vi "Main.vi"() -> ()   [LabVIEW 2012, in "HGF_ApplicationBaseClasses.lvlib" / "HGF_Application.lvclass"]
uses:
  HGF_Application.lvclass
  HGF_BaseClasses/HGF_Factory/HGF_Factory.lvclass
  HGF_BaseClasses/HGF_Event/HGF_Event.lvclass
  HGF_BaseClasses/HGF_Stop/HGF_Stop.lvclass
  HGF_Application.lvclass/HGF_Application.ctl
  HGF_Configuration/HGF_Configuration.lvclass
  HGF_Auxiliary/HGF_Auxiliary.lvlib
  HGF_BaseClasses/HGF_Timing/HGF_Timing.lvclass
  <vilib>/lvdsc/NI_DSC.lvlib
panel:
  in  "HDV":bool
  in  "Alarm and Event Display":refnum<k7>(container)
  in  "read parameters":T1={"Min priority"=0, "Max priority"=1000, "Show Acknowledged alarms?"=FALSE} {"Max priority" max=1000 step=1; "Min priority" max=1000 step=1}
  out "Alarm Summary Data":T2
  out "Time Stamp":timestamp format="%<%H:%M:%S\n%m/%d>T"
  out "Status":string
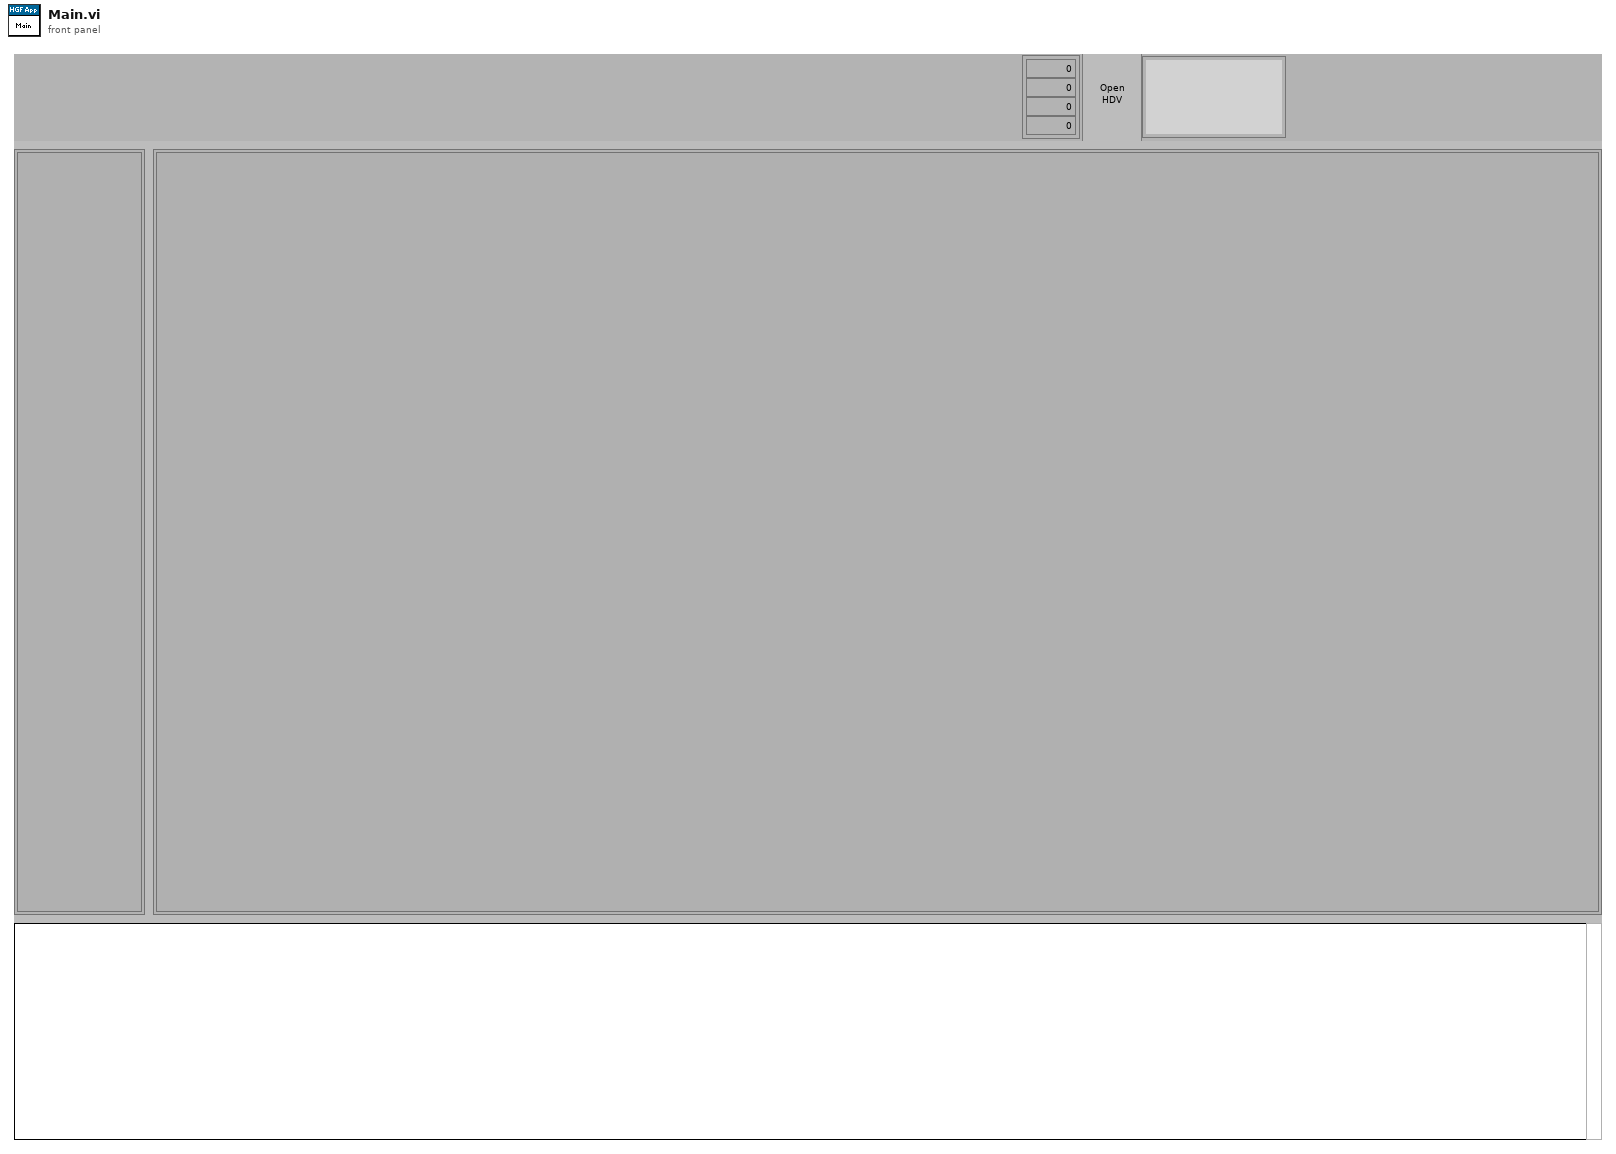
[diagram p1: front panel]
types:
  T1 = cluster{"Min priority":u32, "Max priority":u32, "Show Acknowledged alarms?":bool}
  T2 = cluster{"# active alarms occurrences":i32, "any alarm occurrences?":bool, "# unack alarms occurrences":i32, "any unack alarm occurrences?":bool, "# tags with active alarms":i32, "any tags with alarms?":bool, "# tags with unack alarms":i32, "any tags with unack alarms?":bool}
  T3 = enum32{"invalid app kind", "Development System", "Run Time System", "Student Edition", "Embedded LabVIEW", "Evaluation", "Custom"}
  T4 = cluster{"# active alarms occurrences":i32, "any alarm occurrences?":bool, "# unack alarms occurrences":i32, "any unack alarm occurrences?":bool, "# shared variables with active alarms":i32, "any shared variables with alarms?":bool, "# shared variables with unack alarms":i32, "any shared variables with unack alarms?":bool}
  T5 = cluster{"seconds since 1Jan1904":timestamp, string}
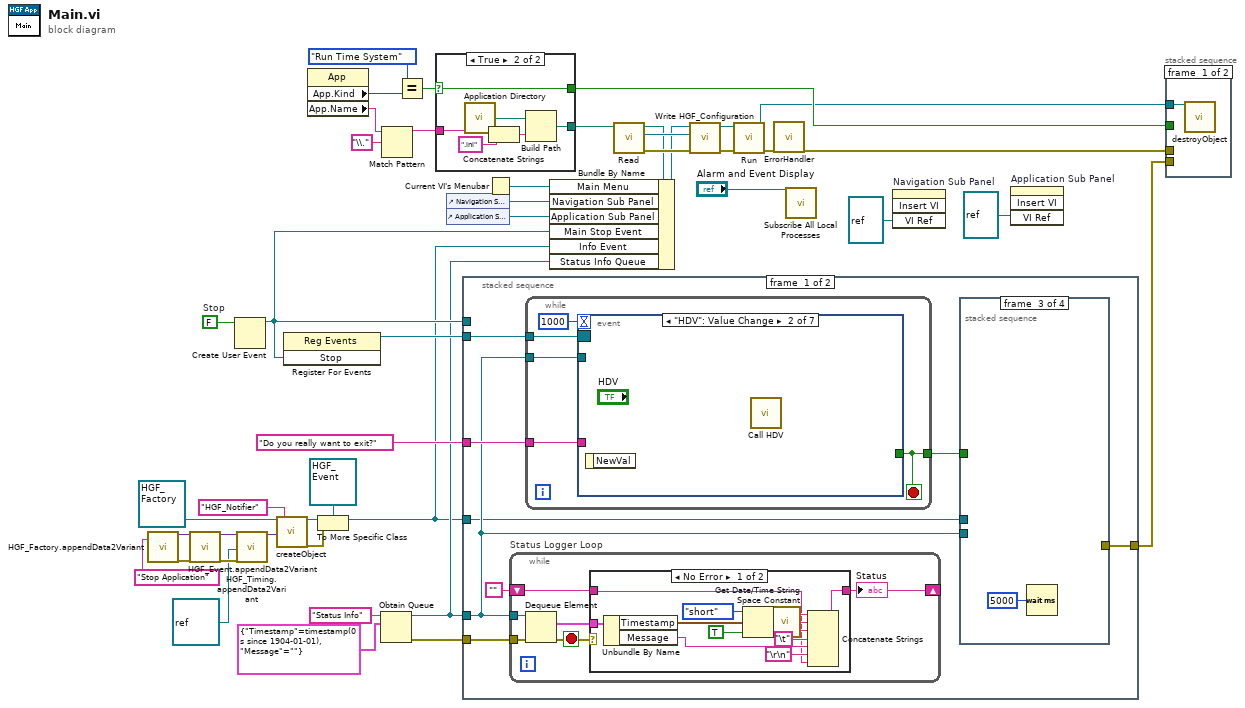
[diagram p0: block diagram]
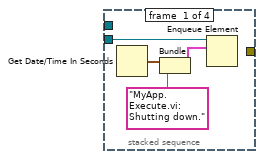
[diagram p2: hidden frame]
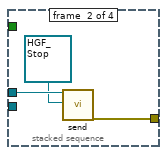
[diagram p3: hidden frame]
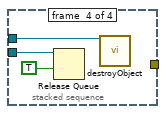
[diagram p4: hidden frame]
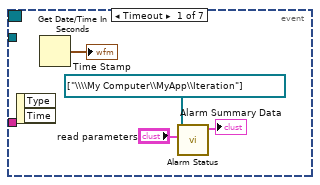
[diagram p6: hidden frame]
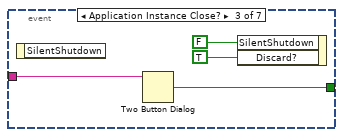
[diagram p7: hidden frame]
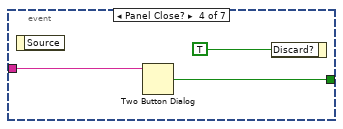
[diagram p8: hidden frame]
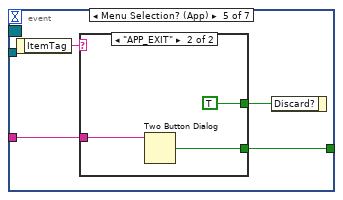
[diagram p9: hidden frame]
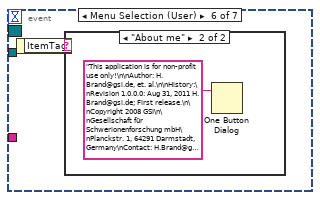
[diagram p11: hidden frame]
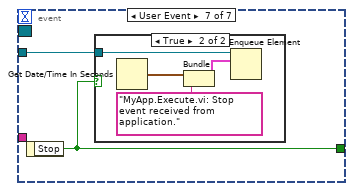
[diagram p13: hidden frame]
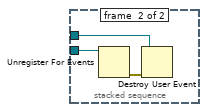
[diagram p15: hidden frame]
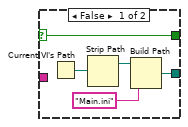
[diagram p16: hidden frame]
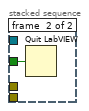
[diagram p17: hidden frame]
diagram:
  w33 = FALSE  # Stop
  n1 = call "HGF_Factory.appendData2Variant.vi"("objectName"="Stop Application") -> ("dup initData"=w20:variant, "error out"=w17:errorcluster)  [unwired: 17 in]
  n2 = call "HGF_Event.appendData2Variant.vi"("initData"=w20, "error in (no error)"=w17) -> ("dup initData"=w19:variant, "error out"=w18:errorcluster)  [unwired: 16 in]
  n3 = Create User Event(user event datatype=w33) -> (user event=w29:refnum<user-event>)  [unwired: 1 in, 1 out]
  n4 = call "HGF_Timing.appendData2Variant.vi"("initData"=w19, "defaultObject"=refnum<class> refnum, "error in (no error)"=w18) -> ("dup initData"=w16:variant)  [unwired: 15 in, 1 out]
  n5 = call "createObject.vi"("HGF_Factory"=refnum<class "HGF_Factory.lvclass"> refnum ("HGF_BaseClasses.lvlib:HGF_Factory.lvclass"), "initializationData"=w16, "className"="HGF_Notifier") -> ("HGF_Object"=w15:refnum<class "HGF_Factory.lvclass">, "error out"=w14:errorcluster)  [unwired: 14 in, 1 out]
  n6 = register-events(w29) -> (reference out=w32:refnum<event-registration>)  [unwired: 2 in, 1 out]
  n7 = property class="App"() -> ("App.Kind"=w37:T3, "App.Name"=w2:string)  [unwired: 2 in, 2 out]
  n8 = To More Specific Class(target class=refnum<class "HGF_Event.lvclass"> refnum ("HGF_BaseClasses.lvlib:HGF_Event.lvclass"), reference=w15, error in=w14) -> (specific class reference=w9:refnum<class "HGF_Event.lvclass">)  [unwired: 1 out]
  n9 = Obtain Queue(name (unnamed)="Status Info", element data type=cluster{"Timestamp":timestamp, "Message":string} {"Timestamp"=timestamp(0 s since 1904-01-01), "Message"=""}) -> (queue out=w10:refnum<queue>, error out=w26:errorcluster)  [unwired: 3 in, 1 out]
  n10 = Match Pattern(string=w2, regular expression="\\.") -> (before substring=w3:string)  [unwired: 1 in, 3 out]
  n11 = Equal?(x=T3."Run Time System" ("Application:Kind"), y=w37) -> (x = y?=w36:bool)
  n12 = case shown="True" w36 {
    selector: w36 -> [w46 w56]
    tunnel: [w47 w54] -> w45
    tunnel: [w46 w56] -> w35
    tunnel: w3 -> [_ w52]
    frame False {
      n13 = Current VI's Path() -> (path=w50:path)
      n14 = Strip Path(path=w50) -> (stripped path=w49:path)  [unwired: 1 out]
      n15 = Build Path(base path=w49, name or relative path="Main.ini") -> (appended path=w47:path)
    }
    frame True {
      n16 = call <vilib>:"Application Directory.vi"() -> ("Application Directory"=w55:path)
      n17 = Concatenate Strings(w52, ".ini" ("name or relative path")) -> (w51:string)
      n18 = Build Path(base path=w55, name or relative path=w51) -> (appended path=w54:path)
    }
  }
  n19 = control-ref of="Navigation Sub Panel"() -> (w8:refnum<vi>)
  n20 = control-ref of="Application Sub Panel"() -> (w7:refnum<vi>)
  n21 = stacked-sequence {
    tunnel: "Do you really want to exit?" ("message") -> [w64 _]
    tunnel: w32 -> [w63 w128]
    tunnel: w29 -> [_ w127]
    tunnel: w10 -> [w60 _]
    tunnel: w26 -> [w62 _]
    tunnel: w9 -> [w58 _]
    tunnel: [w57 _] -> w6
    frame #0 {
      n22 = while "Status Logger Loop" {
        tunnel: w60 -> [w81]
        tunnel: w62 -> [w80]
        shift-right: [w77] -> _
        shift-left: "" -> [w78]
        stop <- w76 stop-if-true
        n23 = Dequeue Element(queue=w81, error in (no error)=w80) -> (element=w79:cluster{"Timestamp":timestamp, "Message":string}, error out=w76:errorcluster)  [unwired: 1 in, 2 out]
        n24 = case shown="No Error" w76 {
          tunnel: w79 -> [w91 _]
          tunnel: w78 -> [w82 w94]
          tunnel: [w83 w94] -> w77
          frame No Error {
            n25 = Unbundle By Name(w91) -> ("Timestamp"=w90:timestamp, "Message"=w86:string)
            n26 = Get Date/Time String(date format (0)=enum16{"short", "long", "abbreviated"}."short", seconds (now)=w90, want seconds? (F)=TRUE) -> (date string=w89:string, time string=w88:string)
            n27 = call <vilib>:"Space Constant.vi"() -> ("String"=w87:string)
            n28 = Concatenate Strings(w89, w87, w88, "\t", w86, "\r\n", w82) -> (w83:string)
          }
          frame Error {
          }
        }
        "Status" <- w77
      }
      n29 = while {
        tunnel: w64 -> [w99]
        tunnel: w63 -> [w98]
        tunnel: [w96] -> w61
        tunnel: w60 -> [w95]
        stop <- w96 stop-if-true
        n30 = event shown="[1] \"HDV\": Value Change" {
          selector: w98 -> [_ _ _ _ _ _ _]
          dyn-events: _ -> [_ _ _ _ _ _ _]
          timeout: 1000 -> [_ _ _ _ _ _ _]
          tunnel: w99 -> [_ _ w105 w109 w113 _ _]
          tunnel: [_ _ w104 w108 w112 _ w120] -> w96
          tunnel: w95 -> [_ _ _ _ _ _ w121]
          event Timeout {
            n31 = event-data() -> ()  [unwired: 1 in, 2 out]
            n32 = Get Date/Time In Seconds() -> (seconds since 1Jan1904=→"Time Stamp":timestamp)
            n33 = call <vilib>:"Alarm Status.vi"("read parameters"="read parameters", "shared variables"=refnum<k21>[] ["\\\\My Computer\\MyApp\\Iteration"]) -> ("alarm summary data"=→"Alarm Summary Data":T4)  [unwired: 8 in, 1 out]
          }
          event "HDV": Value Change {
            n34 = event-data() -> ()  [unwired: 1 in, 1 out]
            n35 = call <vilib>:"Call HDV.vi"() -> ()  [unwired: 14 in, 2 out]
          }
          event Application Instance Close? {
            n36 = event-data() -> ()  [unwired: 1 in, 1 out]
            n37 = Two Button Dialog(message=w105) -> (T button?=w104:bool)  [unwired: 2 in]
            n38 = event-data("SilentShutdown"=FALSE, "Discard?"=TRUE) -> ()  [unwired: 1 in, 1 out]
          }
          event Panel Close? {
            n39 = event-data() -> ()  [unwired: 1 in, 1 out]
            n40 = Two Button Dialog(message=w109) -> (T button?=w108:bool)  [unwired: 2 in]
            n41 = event-data("Discard?"=TRUE) -> ()  [unwired: 1 in, 1 out]
          }
          event Menu Selection? (App) {
            n42 = event-data() -> ("ItemTag"=w114:string)  [unwired: 1 in]
            n43 = case shown="\"APP_EXIT\"" w114 {
              tunnel: w113 -> [_ w117]
              tunnel: [_ w116] -> w112
              tunnel: [_ TRUE] -> w111
              frame "False", Default {
              }
              frame "APP_EXIT" {
                n44 = Two Button Dialog(message=w117) -> (T button?=w116:bool)  [unwired: 2 in]
              }
            }
            n45 = event-data("Discard?"=w111) -> ()  [unwired: 1 in, 1 out]
          }
          event Menu Selection (User) {
            n46 = event-data() -> ("ItemTag"=w118:string)  [unwired: 1 in]
            n47 = case shown="\"About me\"" w118 {
              frame "False", Default {
              }
              frame "About me" {
                n48 = One Button Dialog(message="This application is for non-profit use only!\n\nAuthor: H.Brand@gsi.de, et. al.\n\nHistory:\nRevision 1.0.0.0: Aug 31, 2011 H.Brand@gsi.de; First release.\n\nCopyright 2008 GSI\n\nGesellschaft für Schwerionenforschung mbH\nPlanckstr. 1, 64291 Darmstadt, Germany\nContact: H.Brand@gsi.de or D.Beck@gsi.de\n\nThis file is part of the HGF LVOOP base class library.\n\n    HGF LVOOP base class library is free software: you can redistribute it and/or modify\n    it under the terms of the GNU General Public License as published by\n    the Free Software Foundation, either version 3 of the License, or\n    (at your option) any later version.\n\n    HGF LVOOP base class library is distributed in the hope that it will be useful,\n    but WITHOUT ANY WARRANTY; without even the implied warranty of\n    MERCHANTABILITY or FITNESS FOR A PARTICULAR PURPOSE.  See the\n    GNU General Public License for more details.\n\n    You should have received a copy of the GNU General Public License\n    along with HGF LVOOP base class library.  If not, see http://www.gnu.org/licenses/.") -> ()  [unwired: 1 in, 1 out]
              }
            }
          }
          event User Event {
            n49 = event-data() -> ("Stop"=w120:bool)  [unwired: 1 in]
            n50 = case shown="True" w120 {
              tunnel: w121 -> [_ w125]
              frame False {
              }
              frame True {
                n51 = Get Date/Time In Seconds() -> (seconds since 1Jan1904=w124:timestamp)
                n52 = Bundle("seconds since 1Jan1904"=w124, "MyApp.Execute.vi: Stop event received from application.") -> (w123:T5)  [unwired: 1 in]
                n53 = Enqueue Element(queue=w125, element=w123) -> ()  [unwired: 2 in, 3 out]
              }
            }
          }
        }
      }
      n54 = stacked-sequence {
        tunnel: w60 -> [w65 _ _ w74]
        tunnel: w61 -> [_ _ _ _]
        tunnel: w58 -> [_ w71 _ w73]
        tunnel: [_ w69 _ _] -> w57
        frame #0 {
          n55 = Get Date/Time In Seconds() -> (seconds since 1Jan1904=w66:timestamp)
          n56 = Bundle("seconds since 1Jan1904"=w66, "MyApp.Execute.vi: Shutting down.") -> (w67:T5)  [unwired: 1 in]
          n57 = Enqueue Element(queue=w65, element=w67) -> ()  [unwired: 2 in, 3 out]
        }
        frame #1 {
          n58 = call-dynamic "send.vi"("HGF_Event"=w71, "Object"=refnum<class "HGF_Stop.lvclass"> refnum ("HGF_BaseClasses.lvlib:HGF_Stop.lvclass")) -> ("error out"=w69:errorcluster)  [unwired: 15 in, 2 out]
        }
        frame #2 {
          n59 = Wait (ms)(milliseconds to wait=u32 5000) -> ()  [unwired: 1 out]
        }
        frame #3 {
          n60 = Release Queue(queue=w74, force destroy? (F)=TRUE) -> ()  [unwired: 1 in, 3 out]
          n61 = call "destroyObject.vi"("HGF_Factory"=w73) -> ()  [unwired: 18 in, 1 out]
        }
      }
    }
    frame #1 {
      n62 = Unregister For Events(event registration refnum=w128) -> (error out=w126:errorcluster)  [unwired: 1 in]
      n63 = Destroy User Event(user event=w127, error in=w126) -> ()  [unwired: 1 out]
    }
  }
  n64 = Current VI's Menubar() -> (w1:refnum<k9>)
  n65 = call "Read.vi"("Configuration Filename"=w45) -> ("error out"=w43:errorcluster, "HGF_Configuration out"=w44:refnum<class "HGF_Configuration.lvclass">, "HGF_Application out"=w31:refnum<class "HGF_Application.lvclass">)  [unwired: 7 in, 1 out]
  n66 = Bundle By Name(cluster=w31, "Main Menu"=w1, "Navigation Sub Panel"=w8, "Application Sub Panel"=w7, "Main Stop Event"=w29, "Info Event"=w9, "Status Info Queue"=w10) -> (w30:refnum<class "HGF_Application.lvclass">)
  n67 = call "Write HGF_Configuration.vi"("error in (no error)"=w43, "HGF_Configuration"=w44, "HGF_Application in"=w30) -> ("error out"=w41:errorcluster, "HGF_Application out"=w42:refnum<class "HGF_Application.lvclass">)  [unwired: 7 in]
  n68 = call "Run.vi"("error in (no error)"=w41, "HGF_Application in"=w42) -> ("error out"=w39:errorcluster, "HGF_Application out"=w5:refnum<class "HGF_Application.lvclass">)  [unwired: 8 in]
  n69 = call "ErrorHandler.vi"("error in (no error)"=w39) -> ("error out"=w40:errorcluster)  [unwired: 13 in, 5 out]
  n70 = call <vilib>:"Subscribe All Local Processes.vi"("Alarm & Event Displayer reference"="Alarm and Event Display") -> ()  [unwired: 9 in, 2 out]
  n71 = invoke on="Navigation Sub Panel" class="SubPanel" method="Insert VI"("VI Ref"=refnum<vi> refnum) -> ()  [unwired: 3 in, 4 out]
  n72 = invoke on="Application Sub Panel" class="SubPanel" method="Insert VI"("VI Ref"=refnum<vi> refnum) -> ()  [unwired: 3 in, 4 out]
  n73 = stacked-sequence {
    tunnel: w40 -> [_ _]
    tunnel: w35 -> [_ w130]
    tunnel: w6 -> [_ _]
    tunnel: w5 -> [w129 _]
    frame #0 {
      n74 = call "destroyObject.vi"("HGF_Factory"=w129) -> ()  [unwired: 18 in, 1 out]
    }
    frame #1 {
      n75 = Quit LabVIEW(quit? (T)=w130) -> ()
    }
  }
